vi "filter.get.memory.vi"(11 "filter.data in":T1 {"get.state"."v"."Quantity" format="%.0x"; "get.state"."v"."OrderId" format="%.0x"; "mem.cmd"."ord.2"."v"."Quantity" format="%016x"; "mem.cmd"."ord.2"."v"."OrderId" format="%016x"; "mem.cmd"."ord.1"."v"."Quantity" format="%016x"; "mem.cmd"."ord.1"."v"."OrderId" format="%016x"; "mem.cmd"."ticker"."v"."Symbol" format="%016x"; "mem.cmd"."order.slot.value"."Quantity" format="%016x"; "mem.cmd"."order.slot.value"."OrderId" format="%016x"; "debug"."v"."slot.3" format="%.0x"; "debug"."v"."slot.2" format="%.0x"; "debug"."v"."slot.1" format="%.0x"; "debug"."v"."slot.0" format="%.0x"; "Scratch"."OrderId" format="%016x"; "hash.2"."data.in" format="%.0x"; "hash.2"."crc32.out" format="%.0x"; "hash.1"."data.in" format="%.0x"; "hash.1"."crc32.out" format="%.0x"}) -> (3 "filter.data out":T1 {"get.state"."v"."Quantity" format="%.0x"; "get.state"."v"."OrderId" format="%.0x"; "mem.cmd"."ord.2"."v"."Quantity" format="%016x"; "mem.cmd"."ord.2"."v"."OrderId" format="%016x"; "mem.cmd"."ord.1"."v"."Quantity" format="%016x"; "mem.cmd"."ord.1"."v"."OrderId" format="%016x"; "mem.cmd"."ticker"."v"."Symbol" format="%016x"; "mem.cmd"."order.slot.value"."Quantity" format="%016x"; "mem.cmd"."order.slot.value"."OrderId" format="%016x"; "debug"."v"."slot.3" format="%.0x"; "debug"."v"."slot.2" format="%.0x"; "debug"."v"."slot.1" format="%.0x"; "debug"."v"."slot.0" format="%.0x"; "Scratch"."OrderId" format="%016x"; "hash.2"."data.in" format="%.0x"; "hash.2"."crc32.out" format="%.0x"; "hash.1"."data.in" format="%.0x"; "hash.1"."crc32.out" format="%.0x"})   [LabVIEW 2020]
uses:
  order.slot.ctl
  ticker.slot.ctl
  filter.memory.command.ctl
  filter.states.ctl
  order.slot.hm.ctl
  order.slot.access.ctl
  ticker.slot.access.ctl
  Filter.lvclass
  filter.debug.slot.ctl
  filter.debug.ctl
  filter.data.scratch.ctl
  Market.Data.Common/fpga/orderbook.command.ctl
  Market.Data.Common/fpga/fpganow.common.fpga.lvlib
  filter.data.ctl
  filter.state.slot.ctl
  filter.state.ctl
  Market.Data.Common/fpga/orderbook.command.type.ctl
  filter.hash.ctl
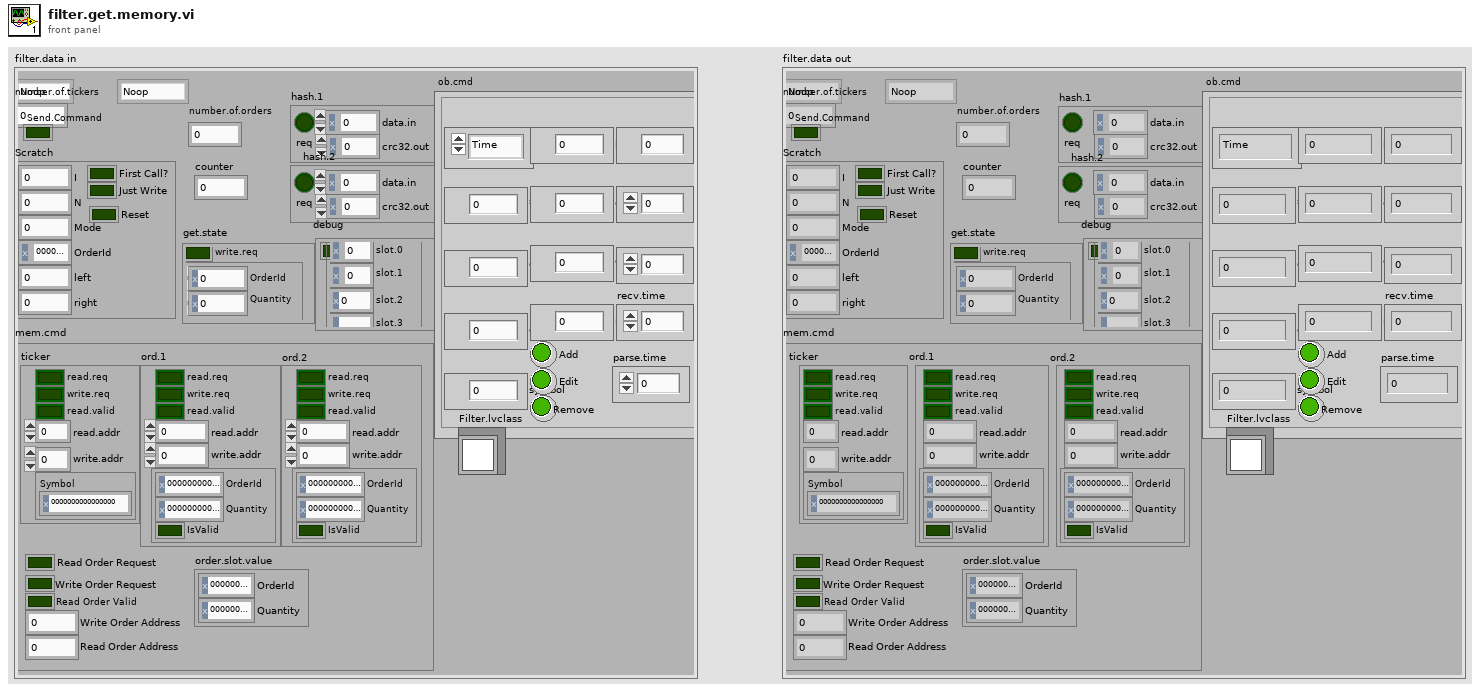
[diagram p1: front panel]
types:
  T1 = typedef "filter.data.ctl" = cluster{"filter.state":T2, "number.of.tickers":u32, "filter.saved.state":T2, "Send.Command":bool, "hash.1":T3, "hash.2":T3, "Scratch":T4, "debug":T5, "mem.cmd":T7, "get.state":T13, "ob.cmd":T15, "number.of.orders":u32, "Filter.lvclass":refnum<class "Filter.lvclass">, "counter":i16}
  T2 = typedef "filter.states.ctl" = enum16{"Noop", "Reset", "Debug", "Configuration", "Wait.for.Command", "Filter.Add", "Filter.Other", "Insert.Order", "Delete Order", "Get.State", "Get.Watchlist", "Get.Memory"}
  T3 = typedef "filter.hash.ctl" = cluster{"req":bool, "data.in":u64, "crc32.out":u32}
  T4 = typedef "filter.data.scratch.ctl" = cluster{"I":u32, "N":u32, "Mode":u32, "OrderId":u64, "First Call?":bool, "Just Write":bool, "left":u32, "right":u32, "Reset":bool}
  T5 = typedef "filter.debug.ctl" = cluster{"write":bool, "v":T6}
  T6 = typedef "filter.debug.slot.ctl" = cluster{"slot.0":u64, "slot.1":u64, "slot.2":u64, "slot.3":u64}
  T7 = typedef "filter.memory.command.ctl" = cluster{"Read Order Request":bool, "Write Order Request":bool, "Read Order Valid":bool, "Write Order Address":u32, "Read Order Address":u32, "order.slot.value":T8, "ticker":T9, "ord.1":T11, "ord.2":T11}
  T8 = typedef "order.slot.ctl" = cluster{"OrderId":u64, "Quantity":u64}
  T9 = typedef "ticker.slot.access.ctl" = cluster{"read.req":bool, "write.req":bool, "read.valid":bool, "read.addr":u32, "write.addr":u32, "v":T10}
  T10 = typedef "ticker.slot.ctl" = cluster{"Symbol":u64}
  T11 = typedef "order.slot.access.ctl" = cluster{"read.req":bool, "write.req":bool, "read.valid":bool, "read.addr":u32, "write.addr":u32, "v":T12}
  T12 = typedef "order.slot.hm.ctl" = cluster{"OrderId":u64, "Quantity":u64, "IsValid":bool}
  T13 = typedef "filter.state.ctl" = cluster{"write.req":bool, "v":T14}
  T14 = typedef "filter.state.slot.ctl" = cluster{"OrderId":u64, "Quantity":u64}
  T15 = typedef "fpganow.common.fpga.lvlib/orderbook.command.ctl" = cluster{"type":T16, "side":u8, "orderId ":u64, "quantity":u32, "symbol":u64, "price":u64, "executed.qty":u32, "canceled.qty":u32, "remaining.qty":u32, "seconds":u64, "nanoseconds":u64, "Add":bool, "Edit":bool, "Remove":bool, "seq no":u32, "recv.time":u64, "parse.time":u64}
  T16 = typedef "fpganow.common.fpga.lvlib/orderbook.command.type.ctl" = enum8{"Time", "AddOrder", "OrderExecuted", "OrderExecutedAtPrice", "ReduceSize", "ModifyOrder", "DeleteOrder", "Get.Everything", "Get.All.Orders", "Get.Top"}
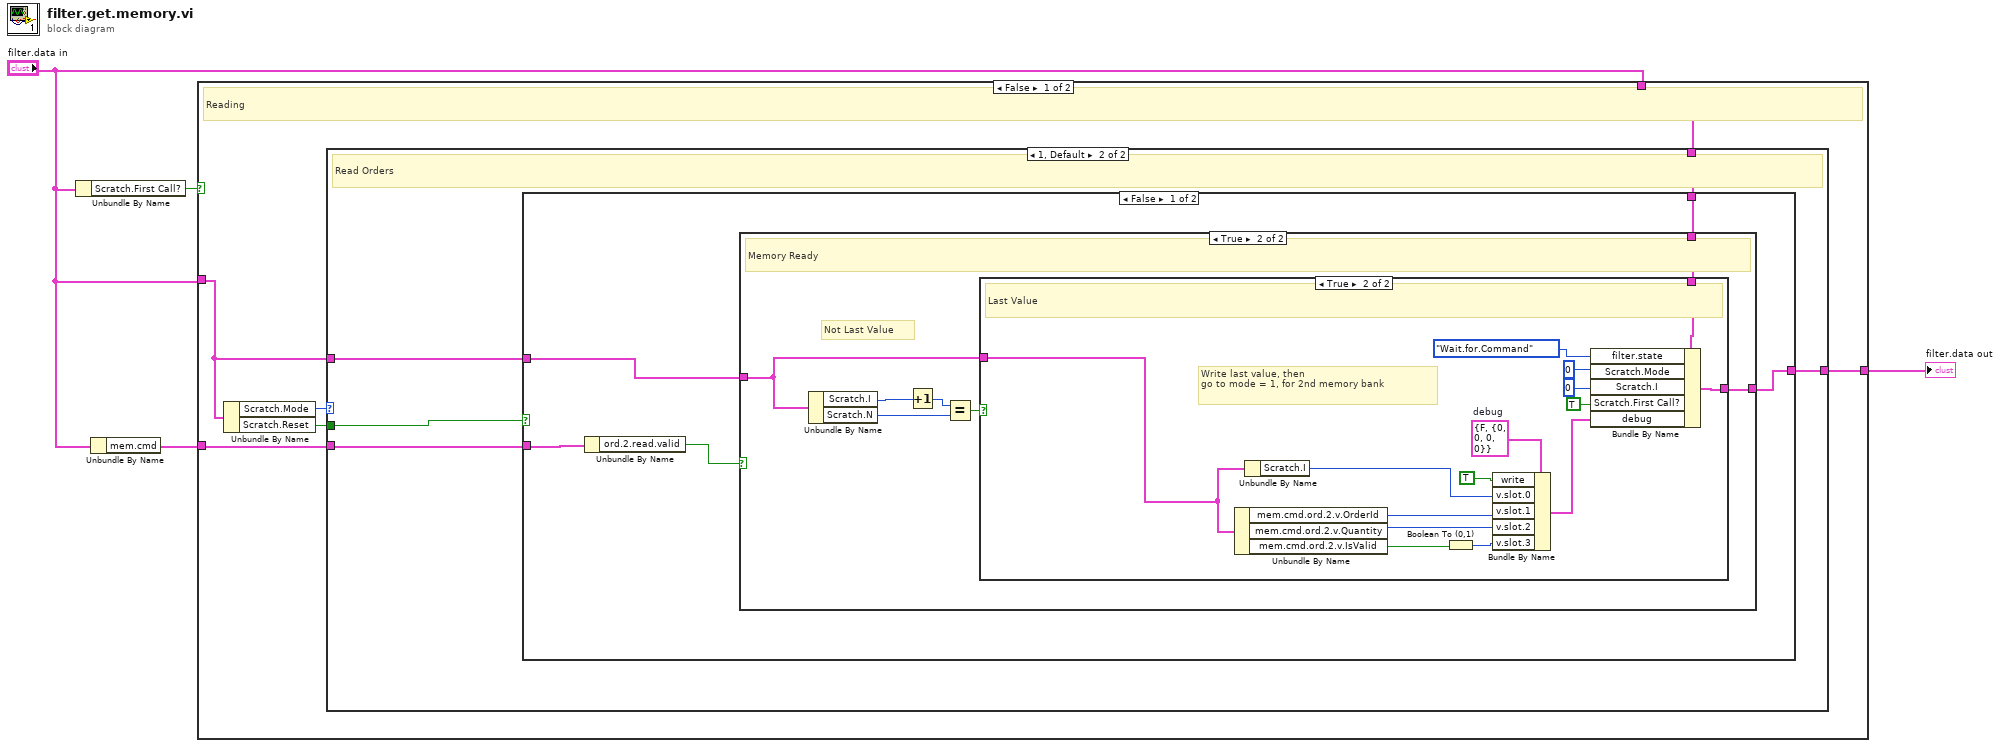
[diagram p0: block diagram]
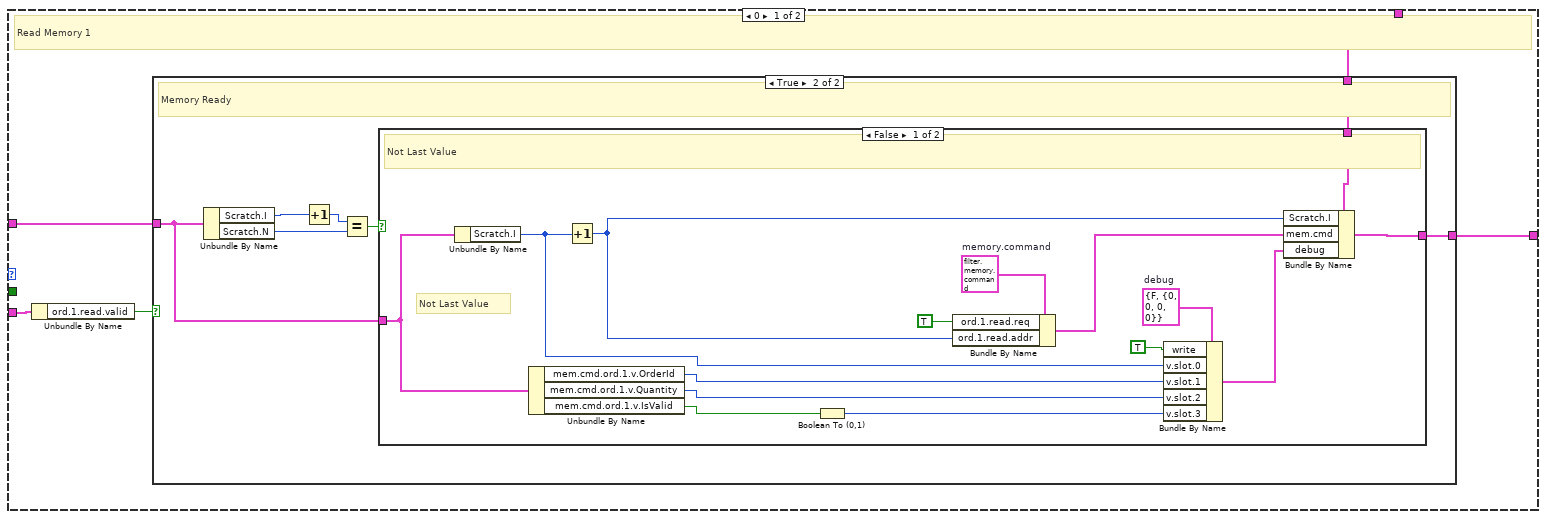
[diagram p2: hidden frame]
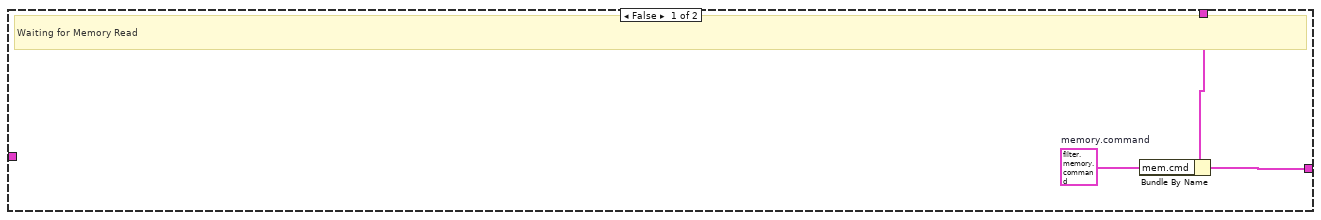
[diagram p3: hidden frame]
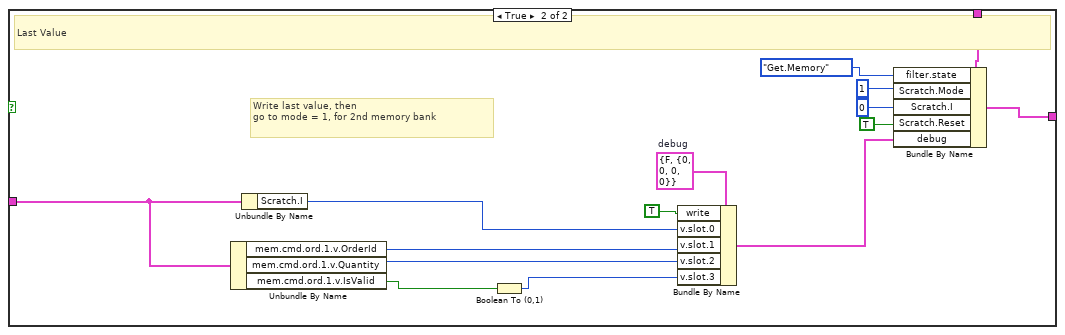
[diagram p4: hidden frame]
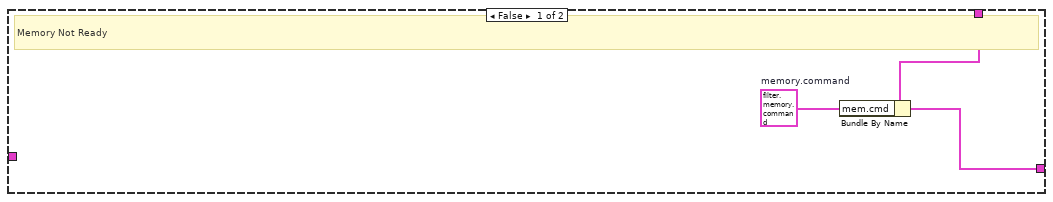
[diagram p5: hidden frame]
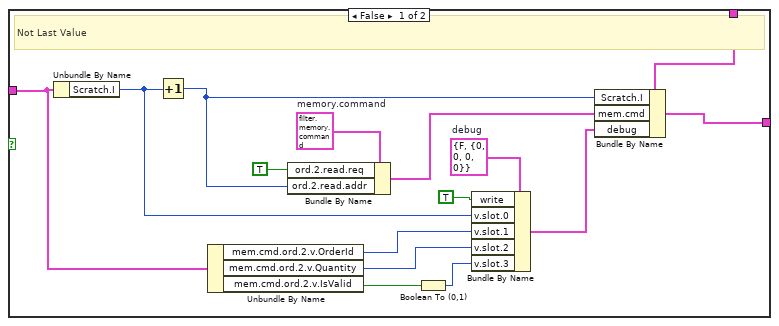
[diagram p6: hidden frame]
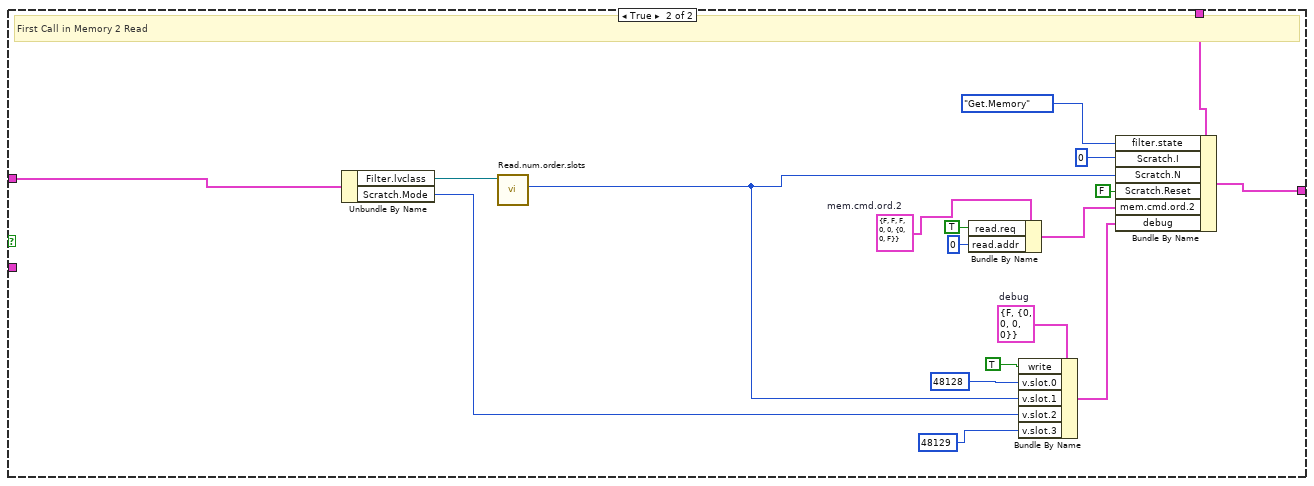
[diagram p7: hidden frame]
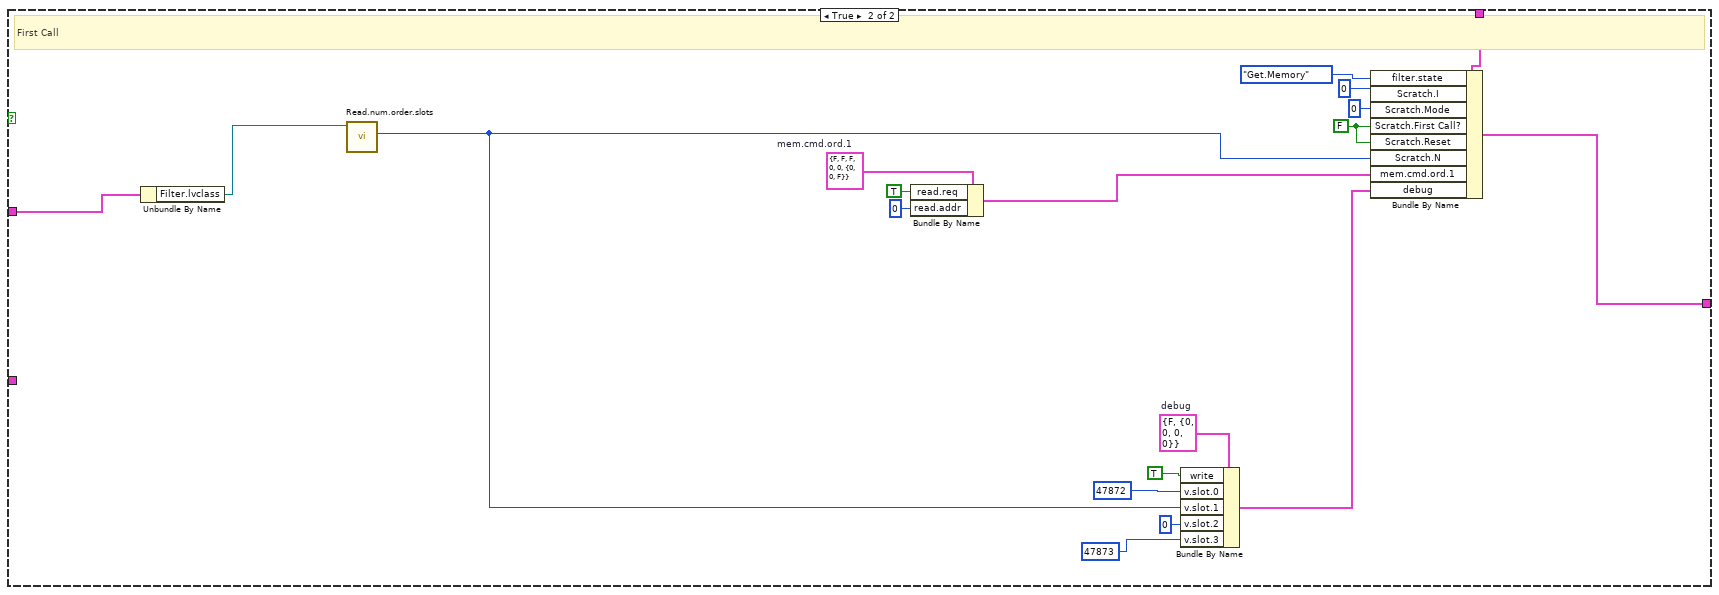
[diagram p8: hidden frame]
diagram:
  n1 = Unbundle By Name("filter.data in") -> ("Scratch.First Call?"=w1:bool)
  n2 = Unbundle By Name("filter.data in") -> ("mem.cmd"=w4:T7)
  n3 = case shown="False" w1 {
    tunnel: "filter.data in" -> [w9 w142]
    tunnel: [w10 w141] -> w2
    tunnel: "filter.data in" -> [w7 w134]
    tunnel: w4 -> [w8 _]
    frame False {
      # "Reading"
      n4 = Unbundle By Name(w7) -> ("Scratch.Mode"=w6:u32, "Scratch.Reset"=w5:bool)
      n5 = case shown="1, Default" w6 {
        tunnel: [w15 w60] -> w10
        tunnel: w9 -> [w14 w59]
        tunnel: w8 -> [w12 w58]
        tunnel: w7 -> [w11 w57]
        tunnel: w5 -> [_ w56]
        frame 0 {
          # "Read Memory 1"
          n6 = Unbundle By Name(w12) -> ("ord.1.read.valid"=w13:bool)
          n7 = case shown="True" w13 {
            tunnel: [w16 w19] -> w15
            tunnel: w14 -> [w18 w20]
            tunnel: w11 -> [_ w21]
            frame False {
              w17 = T7 {"Read Order Request"=FALSE, "Write Order Request"=FALSE, "Read Order Valid"=FALSE, "Write Order Address"=0, "Read Order Address"=0, "order.slot.value"={"OrderId"=0, "Quantity"=0}, "ticker"={"read.req"=FALSE, "write.req"=FALSE, "read.valid"=FALSE, "read.addr"=0, "write.addr"=0, "v"={"Symbol"=0}}, "ord.1"={"read.req"=FALSE, "write.req"=FALSE, "read.valid"=FALSE, "read.addr"=0, "write.addr"=0, "v"={"OrderId"=0, "Quantity"=0, "IsValid"=FALSE}}, "ord.2"={"read.req"=FALSE, "write.req"=FALSE, "read.valid"=FALSE, "read.addr"=0, "write.addr"=0, "v"={"OrderId"=0, "Quantity"=0, "IsValid"=FALSE}}}  # memory.command
              # "Waiting for Memory Read"
              n8 = Bundle By Name(cluster=w18, "mem.cmd"=w17) -> (w16:T1)
            }
            frame True {
              # "Memory Ready"
              n9 = Unbundle By Name(w21) -> ("Scratch.I"=w25:u32, "Scratch.N"=w23:u32)
              n10 = Increment(x=w25) -> (x+1=w24:u32)
              n11 = Equal?(x=w24, y=w23) -> (x = y?=w22:bool)
              n12 = case shown="False" w22 {
                tunnel: w21 -> [w37 w44]
                tunnel: w20 -> [w34 w55]
                tunnel: [w40 w54] -> w19
                frame False {
                  w32 = T5 {"write"=FALSE, "v"={"slot.0"=0, "slot.1"=0, "slot.2"=0, "slot.3"=0}}  # debug
                  w39 = T7 {"Read Order Request"=FALSE, "Write Order Request"=FALSE, "Read Order Valid"=FALSE, "Write Order Address"=0, "Read Order Address"=0, "order.slot.value"={"OrderId"=0, "Quantity"=0}, "ticker"={"read.req"=FALSE, "write.req"=FALSE, "read.valid"=FALSE, "read.addr"=0, "write.addr"=0, "v"={"Symbol"=0}}, "ord.1"={"read.req"=FALSE, "write.req"=FALSE, "read.valid"=FALSE, "read.addr"=0, "write.addr"=0, "v"={"OrderId"=0, "Quantity"=0, "IsValid"=FALSE}}, "ord.2"={"read.req"=FALSE, "write.req"=FALSE, "read.valid"=FALSE, "read.addr"=0, "write.addr"=0, "v"={"OrderId"=0, "Quantity"=0, "IsValid"=FALSE}}}  # memory.command
                  # "Not Last Value"
                  # "Not Last Value"
                  n13 = Unbundle By Name(w37) -> ("Scratch.I"=w30:u32)
                  n14 = Unbundle By Name(w37) -> ("mem.cmd.ord.1.v.OrderId"=w29:u64, "mem.cmd.ord.1.v.Quantity"=w28:u64, "mem.cmd.ord.1.v.IsValid"=w27:bool)
                  n15 = Increment(x=w30) -> (x+1=w35:u32)
                  n16 = Boolean To (0,1)(Boolean=w27) -> (0, 1=w26:i16)
                  n17 = Bundle By Name(cluster=w39, "ord.1.read.req"=TRUE ("Read.Request"), "ord.1.read.addr"=w35) -> (w38:T7)
                  n18 = Bundle By Name(cluster=w32, "write"=TRUE ("write.req"), "v.slot.0"=w30, "v.slot.1"=w29, "v.slot.2"=w28, "v.slot.3"=w26) -> (w31:T5)
                  n19 = Bundle By Name(cluster=w34, "Scratch.I"=w35, "mem.cmd"=w38, "debug"=w31) -> (w40:T1)
                }
                frame True {
                  w50 = T5 {"write"=FALSE, "v"={"slot.0"=0, "slot.1"=0, "slot.2"=0, "slot.3"=0}}  # debug
                  # "Write last value, then\ngo to mode = 1, for 2nd memory bank"
                  # "Last Value"
                  n20 = Unbundle By Name(w44) -> ("mem.cmd.ord.1.v.OrderId"=w45:u64, "mem.cmd.ord.1.v.Quantity"=w46:u64, "mem.cmd.ord.1.v.IsValid"=w48:bool)
                  n21 = Unbundle By Name(w44) -> ("Scratch.I"=w43:u32)
                  n22 = Boolean To (0,1)(Boolean=w48) -> (0, 1=w47:i16)
                  n23 = Bundle By Name(cluster=w50, "write"=TRUE ("write.req"), "v.slot.0"=w43, "v.slot.1"=w45, "v.slot.2"=w46, "v.slot.3"=w47) -> (w49:T5)
                  n24 = Bundle By Name(cluster=w55, "filter.state"=filter.states."Get.Memory" ("f"), "Scratch.Mode"=u32 1, "Scratch.I"=u32 0, "Scratch.Reset"=TRUE ("Scratch.First Call?"), "debug"=w49) -> (w54:T1)
                }
              }
            }
          }
        }
        frame 1, Default {
          # "Read Orders"
          n25 = case shown="False" w56 {
            tunnel: [w65 w119] -> w60
            tunnel: w59 -> [w64 w120]
            tunnel: w58 -> [w62 _]
            tunnel: w57 -> [w61 w117]
            frame False {
              n26 = Unbundle By Name(w62) -> ("ord.2.read.valid"=w63:bool)
              n27 = case shown="True" w63 {
                tunnel: [w66 w69] -> w65
                tunnel: w64 -> [w68 w70]
                tunnel: w61 -> [_ w71]
                frame False {
                  w67 = T7 {"Read Order Request"=FALSE, "Write Order Request"=FALSE, "Read Order Valid"=FALSE, "Write Order Address"=0, "Read Order Address"=0, "order.slot.value"={"OrderId"=0, "Quantity"=0}, "ticker"={"read.req"=FALSE, "write.req"=FALSE, "read.valid"=FALSE, "read.addr"=0, "write.addr"=0, "v"={"Symbol"=0}}, "ord.1"={"read.req"=FALSE, "write.req"=FALSE, "read.valid"=FALSE, "read.addr"=0, "write.addr"=0, "v"={"OrderId"=0, "Quantity"=0, "IsValid"=FALSE}}, "ord.2"={"read.req"=FALSE, "write.req"=FALSE, "read.valid"=FALSE, "read.addr"=0, "write.addr"=0, "v"={"OrderId"=0, "Quantity"=0, "IsValid"=FALSE}}}  # memory.command
                  # "Memory Not Ready"
                  n28 = Bundle By Name(cluster=w68, "mem.cmd"=w67) -> (w66:T1)
                }
                frame True {
                  # "Not Last Value"
                  # "Memory Ready"
                  n29 = Unbundle By Name(w71) -> ("Scratch.I"=w75:u32, "Scratch.N"=w73:u32)
                  n30 = Increment(x=w75) -> (x+1=w74:u32)
                  n31 = Equal?(x=w74, y=w73) -> (x = y?=w72:bool)
                  n32 = case shown="True" w72 {
                    tunnel: w71 -> [w87 w91]
                    tunnel: w70 -> [w85 w92]
                    tunnel: [w90 w93] -> w69
                    frame False {
                      w82 = T5 {"write"=FALSE, "v"={"slot.0"=0, "slot.1"=0, "slot.2"=0, "slot.3"=0}}  # debug
                      w89 = T7 {"Read Order Request"=FALSE, "Write Order Request"=FALSE, "Read Order Valid"=FALSE, "Write Order Address"=0, "Read Order Address"=0, "order.slot.value"={"OrderId"=0, "Quantity"=0}, "ticker"={"read.req"=FALSE, "write.req"=FALSE, "read.valid"=FALSE, "read.addr"=0, "write.addr"=0, "v"={"Symbol"=0}}, "ord.1"={"read.req"=FALSE, "write.req"=FALSE, "read.valid"=FALSE, "read.addr"=0, "write.addr"=0, "v"={"OrderId"=0, "Quantity"=0, "IsValid"=FALSE}}, "ord.2"={"read.req"=FALSE, "write.req"=FALSE, "read.valid"=FALSE, "read.addr"=0, "write.addr"=0, "v"={"OrderId"=0, "Quantity"=0, "IsValid"=FALSE}}}  # memory.command
                      # "Not Last Value"
                      n33 = Unbundle By Name(w87) -> ("Scratch.I"=w78:u32)
                      n34 = Increment(x=w78) -> (x+1=w84:u32)
                      n35 = Unbundle By Name(w87) -> ("mem.cmd.ord.2.v.OrderId"=w79:u64, "mem.cmd.ord.2.v.Quantity"=w80:u64, "mem.cmd.ord.2.v.IsValid"=w77:bool)
                      n36 = Bundle By Name(cluster=w89, "ord.2.read.req"=TRUE ("Read.Request"), "ord.2.read.addr"=w84) -> (w88:T7)
                      n37 = Boolean To (0,1)(Boolean=w77) -> (0, 1=w76:i16)
                      n38 = Bundle By Name(cluster=w82, "write"=TRUE ("write.req"), "v.slot.0"=w78, "v.slot.1"=w79, "v.slot.2"=w80, "v.slot.3"=w76) -> (w81:T5)
                      n39 = Bundle By Name(cluster=w85, "Scratch.I"=w84, "mem.cmd"=w88, "debug"=w81) -> (w90:T1)
                    }
                    frame True {
                      w102 = T5 {"write"=FALSE, "v"={"slot.0"=0, "slot.1"=0, "slot.2"=0, "slot.3"=0}}  # debug
                      # "Write last value, then\ngo to mode = 1, for 2nd memory bank"
                      # "Last Value"
                      n40 = Unbundle By Name(w91) -> ("mem.cmd.ord.2.v.OrderId"=w97:u64, "mem.cmd.ord.2.v.Quantity"=w98:u64, "mem.cmd.ord.2.v.IsValid"=w100:bool)
                      n41 = Unbundle By Name(w91) -> ("Scratch.I"=w96:u32)
                      n42 = Boolean To (0,1)(Boolean=w100) -> (0, 1=w99:i16)
                      n43 = Bundle By Name(cluster=w102, "write"=TRUE ("write.req"), "v.slot.0"=w96, "v.slot.1"=w97, "v.slot.2"=w98, "v.slot.3"=w99) -> (w101:T5)
                      n44 = Bundle By Name(cluster=w92, "filter.state"=filter.states."Wait.for.Command" ("f"), "Scratch.Mode"=u32 0, "Scratch.I"=u32 0, "Scratch.First Call?"=TRUE, "debug"=w101) -> (w93:T1)
                    }
                  }
                }
              }
            }
            frame True {
              w114 = T5 {"write"=FALSE, "v"={"slot.0"=0, "slot.1"=0, "slot.2"=0, "slot.3"=0}}  # debug
              w121 = T11 {"read.req"=FALSE, "write.req"=FALSE, "read.valid"=FALSE, "read.addr"=0, "write.addr"=0, "v"={"OrderId"=0, "Quantity"=0, "IsValid"=FALSE}}  # mem.cmd.ord.2
              # "First Call in Memory 2 Read"
              n45 = Unbundle By Name(w117) -> ("Filter.lvclass"=w116:refnum<class "Filter.lvclass">, "Scratch.Mode"=w107:u32)
              n46 = call-dynamic "Read.num.order.slots.vi"("Filter in"=w116) -> ("num.order.slots"=w108:u32)  [unwired: 8 in, 2 out]
              n47 = Bundle By Name(cluster=w121, "read.req"=TRUE, "read.addr"=u32 0) -> (w110:T11)
              n48 = Bundle By Name(cluster=w114, "write"=TRUE ("write.req"), "v.slot.0"=u64 48128, "v.slot.1"=w108, "v.slot.2"=w107, "v.slot.3"=u64 48129 ("v.slot.0")) -> (w109:T5)
              n49 = Bundle By Name(cluster=w120, "filter.state"=filter.states."Get.Memory", "Scratch.I"=u32 0, "Scratch.N"=w108, "Scratch.Reset"=FALSE, "mem.cmd.ord.2"=w110, "debug"=w109) -> (w119:T1)
            }
          }
        }
      }
    }
    frame True {
      w132 = T5 {"write"=FALSE, "v"={"slot.0"=0, "slot.1"=0, "slot.2"=0, "slot.3"=0}}  # debug
      w138 = T11 {"read.req"=FALSE, "write.req"=FALSE, "read.valid"=FALSE, "read.addr"=0, "write.addr"=0, "v"={"OrderId"=0, "Quantity"=0, "IsValid"=FALSE}}  # mem.cmd.ord.1
      w124 = FALSE ("Scratch.First Call?")
      # "First Call"
      n50 = Unbundle By Name(w134) -> ("Filter.lvclass"=w133:refnum<class "Filter.lvclass">)
      n51 = call-dynamic "Read.num.order.slots.vi"("Filter in"=w133) -> ("num.order.slots"=w130:u32)  [unwired: 8 in, 2 out]
      n52 = Bundle By Name(cluster=w138, "read.req"=TRUE, "read.addr"=u32 0) -> (w128:T11)
      n53 = Bundle By Name(cluster=w132, "write"=TRUE ("write.req"), "v.slot.0"=u64 47872, "v.slot.1"=w130, "v.slot.2"=u64 0, "v.slot.3"=u64 47873 ("v.slot.0")) -> (w129:T5)
      n54 = Bundle By Name(cluster=w142, "filter.state"=filter.states."Get.Memory", "Scratch.I"=u32 0, "Scratch.Mode"=u32 0, "Scratch.First Call?"=w124, "Scratch.Reset"=w124, "Scratch.N"=w130, "mem.cmd.ord.1"=w128, "debug"=w129) -> (w141:T1)
    }
  }
  "filter.data out" <- w2
